vi "read_4ch_fake.vi"(8 "previous value ch1":bool, 11 "previous value ch0":bool) -> (0 "Inputl1":bool, 2 "read output":T1, 3 "Input0":bool)   [LabVIEW 2010]
uses:
  common_typedefs/channels_cluster.ctl
  <vilib>/eio/EIONode/EIONode.xnode
  <vilib>/rvi/eio/nirviEIOImplementation/nirviEIOImplementation.xnode
  <vilib>/rvi/eio/common/nirviEmuClasses.ctl
  <vilib>/rvi/eio/common/nirviEmuTemplateMethod_noerrors.vi
panel:
  out "s? t:f 2":u32
  out "s? t:f":u32
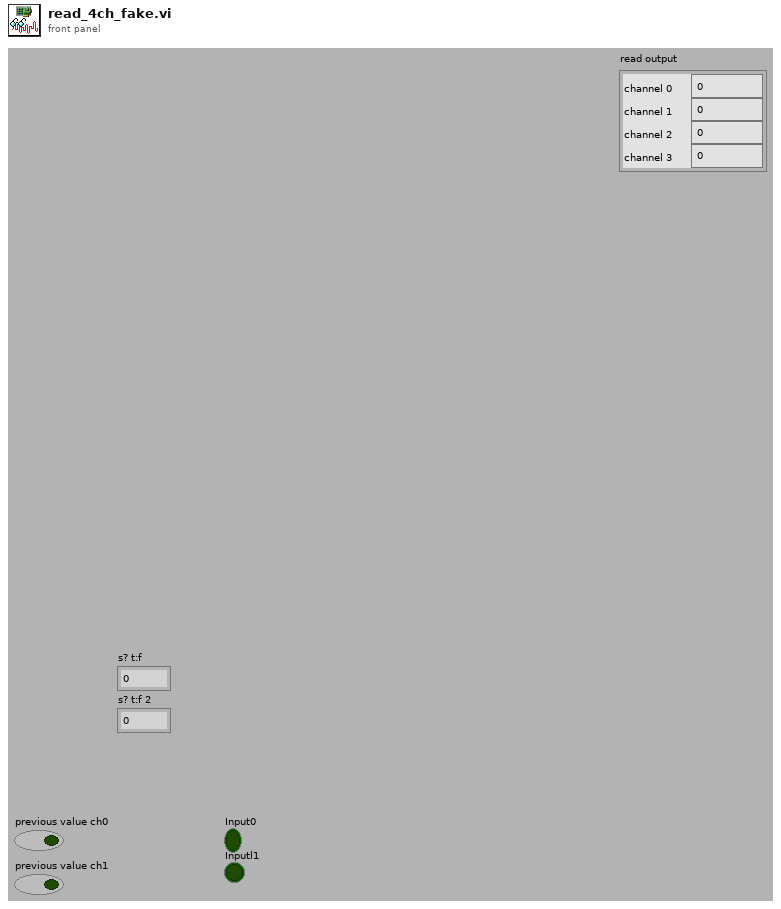
[diagram p1: front panel]
types:
  T1 = typedef "channels_cluster.ctl" = cluster{"channel 0":u32, "channel 1":u32, "channel 2":u32, "channel 3":u32}
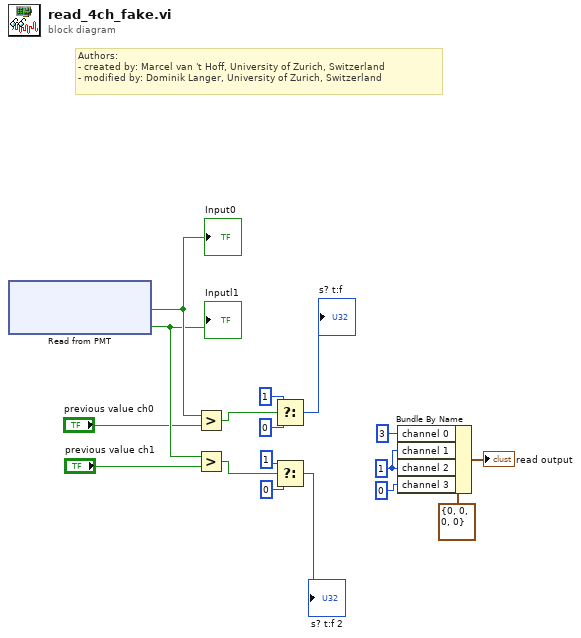
[diagram p0: block diagram]
diagram:
  w1 = u32 1 ("channel 2")
  # "Authors: \n- created by: Marcel van 't Hoff, University of Zurich, Switzerland\n- modified by: Dominik Langer, University of Zurich, Switzerland"
  n1 = xnode "Read from PMT"() -> ("Connector1/DIO23"=w15:bool, "Connector1/DIO1"=w14:bool)  [unwired: 2 in, 2 out]
  "Input0" <- w15
  "Inputl1" <- w14
  n2 = Greater?(x=w15, y="previous value ch0") -> (0:w7:bool)
  n3 = Greater?(x=w14, y="previous value ch1") -> (0:w6:bool)
  n4 = Select(t=u32 1, s=w7, f=u32 0) -> (s? t:f=→"s? t:f":u32)
  n5 = Select(t=u32 1, s=w6, f=u32 0) -> (s? t:f=→"s? t:f 2":u32)
  n6 = Bundle By Name(cluster=T1 {"channel 0"=0, "channel 1"=0, "channel 2"=0, "channel 3"=0} ("channel offsets 3"), "channel 0"=u32 3, "channel 1"=w1, "channel 2"=w1, "channel 3"=u32 0) -> (→"read output":T1)
